vi "Read Test Stand.vi"(8 "error in (no error)":errorcluster, 11 "Run DAC Front Panel in":refnum<class "Run DAC Front Panel.lvclass">) -> (0 "error out":errorcluster, 2 "Generic Test Stand.lvclass":refnum<class "Generic Test Stand.lvclass">, 3 "Run DAC Front Panel out":refnum<class "Run DAC Front Panel.lvclass">)   [LabVIEW 2019, in "DAC Process.lvlib" / "Run DAC Front Panel.lvclass"]
uses:
  Run DAC Front Panel.lvclass
  Generic Test Stand/Generic Test Stand.lvclass
  Run DAC Front Panel.lvclass/Run DAC Front Panel.ctl
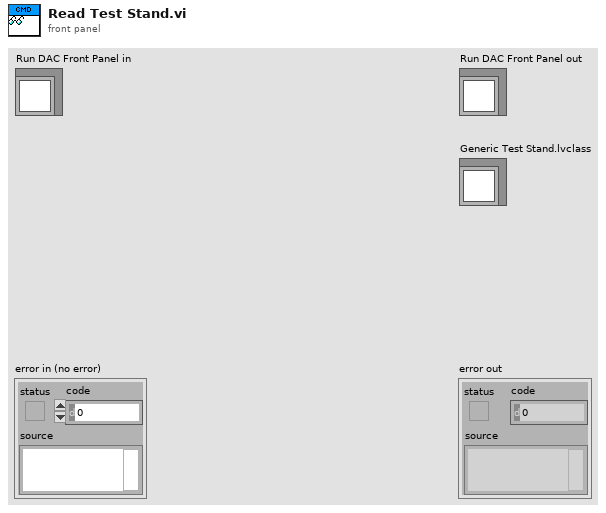
[diagram p1: front panel]
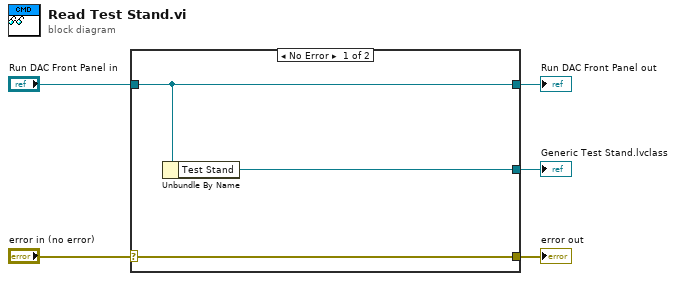
[diagram p0: block diagram]
diagram:
  n1 = case shown="No Error" "error in (no error)" {
    selector: "error in (no error)" -> [w8 w9]
    tunnel: [w8 w9] -> w4
    tunnel: [w7 w10] -> w2
    tunnel: "Run DAC Front Panel in" -> [w7 w10]
    tunnel: [w6 _] -> w1
    frame No Error {
      n2 = Unbundle By Name(w7) -> ("Test Stand"=w6:refnum<class "Generic Test Stand.lvclass">)
    }
    frame Error {
    }
  }
  "error out" <- w4
  "Run DAC Front Panel out" <- w2
  "Generic Test Stand.lvclass" <- w1
